vi "delete_document.vi"(11 "did":string) -> (2 "path":string, 3 "Method":string)   [LabVIEW 2019]
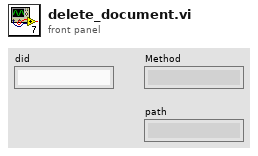
[diagram p1: front panel]
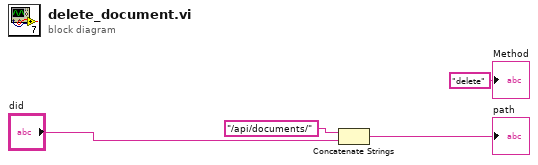
[diagram p0: block diagram]
diagram:
  n1 = Concatenate Strings("/api/documents/" ("payload"), "did") -> (→"path":string)
  "Method" <- "delete" ("Method")
